vi "F Dwf Analog In Status Data2.vi"(6 "cdData":i32, 7 "idxData":i32, 8 "error in (no error)":errorcluster, 9 "rgdVoltData":dbl, 10 "idxChannel":i32, 11 "hdwf":i32) -> (0 "error out":errorcluster, 1 "rgdVoltData out":dbl, 3 "function return":i32)   [LabVIEW 2021, in "Olasdwf.lvlib"]
doc: "DWFAPI int FDwfAnalogInStatusData2(HDWF hdwf, int idxChannel, double *rgdVoltData, int idxData, int cdData);"
uses:
  Olasdwf.lvlib
  Windows/System32/dwf.dll
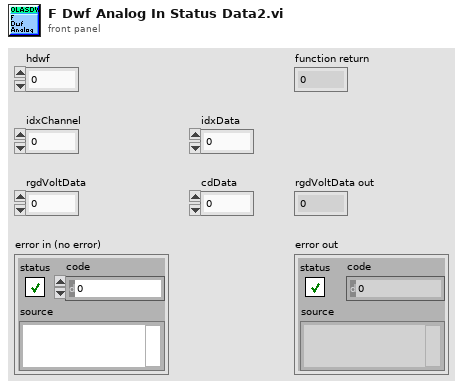
[diagram p1: front panel]
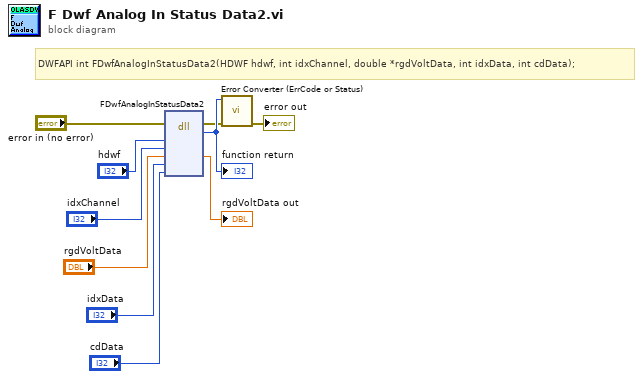
[diagram p0: block diagram]
diagram:
  # "DWFAPI int FDwfAnalogInStatusData2(HDWF hdwf, int idxChannel, double *rgdVoltData, int idxData, int cdData);"
  n1 = dll-call lib="/Windows/System32/dwf.*" fn="FDwfAnalogInStatusData2"(error in="error in (no error)", "hdwf"="hdwf", "idxChannel"="idxChannel", "rgdVoltData"="rgdVoltData", "idxData"="idxData", "cdData"="cdData") -> (error out=w2:errorcluster, w10:i32, "rgdVoltData"=→"rgdVoltData out":dbl)  [unwired: 6 in, 1 out]
  "function return" <- w10
  n2 = call "Error Converter (ErrCode or Status).vi"("error in (no error)"=w2, "error code"=w10) -> ("error out"=→"error out":errorcluster)  [unwired: 9 in]
